vi "ControlsWOOD.vi"() -> ()   [LabVIEW 2016]
uses:
  Typedefs/Sensor Status.ctl
  Modules/Boat/PID Gain.ctl
  Modules/Boat/PID Schedule Entry.ctl
  UI Utilities/ui_states.ctl
  <vilib>/Utility/miscctls.llb/LVPointTypeDef.ctl
  <vilib>/Utility/miscctls.llb/LVPositionTypeDef.ctl
  Messages/autogenerated_vis/receive/mc_receive_state_message.vi
  Minion Core/Minion Core.lvlibp
panel:
  in  "Target":dbl[](array[numeric])
  in  "Main Tabs":T1(tab)
  in  "Navigation Algorithm\nPrimary   -   Fine Manuvering":bool
  out "Back Thrust":dbl(slide) scale=0.0..1.0
  out "?":dbl(slide)
  out "Back Direction":dbl(knob) scale=-1.0..1.0
  out "Front Thrust":dbl(slide) scale=0.0..1.0
  out "?":dbl(slide)
  out "Front Direction":dbl(knob) scale=-1.0..1.0
  in  "Popup Window":bool
  in  "Manage Example":bool
  out "Sensor Status":T2[](array[typedef]) {"Active ID" format="%x"}
  in  "MBED Serial Port":refnum<visa-resource-name>
  out "The String output to mbed":string
  in  "RC(F) Auto(T)":bool
  in  "reinitialize? (F)":bool
  in  "Front Turn Assist Thrust":T3={"Control"={"Mode?"=TRUE, "Active?"=TRUE, "Manual"=0.0}, "PID Schedule"=[], "Input Rate"=0.0, "Output Rate"=0.0, "Filter Input?"=TRUE} {"PID Schedule"."Input Range"."High" format="%.2f"; "PID Schedule"."Input Range"."Low" format="%.2f"; "PID Schedule"."Output Range"."Low" format="%.3f"; "PID Schedule"."Output Range"."High" format="%.3f"; "PID Schedule"."Linearity" format="%#_13g"; "PID Schedule"."PID Gains"."Feedforward"."c" format="%.3f"; "PID Schedule"."PID Gains"."Feedforward"."b" format="%.3f"; "PID Schedule"."PID Gains"."Feedforward"."a" format="%.3f"; "PID Schedule"."PID Gains"."Adv. Gains"."Gamma" format="%.3f"; "PID Schedule"."PID Gains"."Adv. Gains"."Beta" format="%.3f"; "PID Schedule"."PID Gains"."Adv. Gains"."Alpha" format="%.3f"; "PID Schedule"."PID Gains"."Standard Gains"."Kp" format="%.3f"; "PID Schedule"."PID Gains"."Standard Gains"."Ki" format="%.3f"; "PID Schedule"."PID Gains"."Standard Gains"."Kd" format="%.3f"; "Control"."Manual" format="%#_13g"}
  in  "Back Thrust":dbl(slide) scale=0.0..1.0
  in  "Back Steering":T3={"Control"={"Mode?"=TRUE, "Active?"=TRUE, "Manual"=0.0}, "PID Schedule"=[], "Input Rate"=0.0, "Output Rate"=0.0, "Filter Input?"=TRUE} {"PID Schedule"."Input Range"."High" format="%.2f"; "PID Schedule"."Input Range"."Low" format="%.2f"; "PID Schedule"."Output Range"."Low" format="%.3f"; "PID Schedule"."Output Range"."High" format="%.3f"; "PID Schedule"."Linearity" format="%#_13g"; "PID Schedule"."PID Gains"."Feedforward"."c" format="%.3f"; "PID Schedule"."PID Gains"."Feedforward"."b" format="%.3f"; "PID Schedule"."PID Gains"."Feedforward"."a" format="%.3f"; "PID Schedule"."PID Gains"."Adv. Gains"."Gamma" format="%.3f"; "PID Schedule"."PID Gains"."Adv. Gains"."Beta" format="%.3f"; "PID Schedule"."PID Gains"."Adv. Gains"."Alpha" format="%.3f"; "PID Schedule"."PID Gains"."Standard Gains"."Kp" format="%.3f"; "PID Schedule"."PID Gains"."Standard Gains"."Ki" format="%.3f"; "PID Schedule"."PID Gains"."Standard Gains"."Kd" format="%.3f"; "Control"."Manual" format="%#_13g"}
  in  "RC(F) Auto(T)":bool=TRUE
  in  "reinitialize? (F)":bool
  in  "Turbo\nThrust":dbl(slide) scale=0.0..1.0
  in  "Distance\nMinimum for\nTurbo (m)":dbl
  in  "Heading Error\nMaximum for \nTurbo (rad)":dbl
  in  "RC(F) Auto(T)":bool
  in  "reinitialize? (F)":bool
  in  "RC(F) Auto(T)":bool
  in  "reinitialize? (F)":bool
  in  "Desired Boat Orientation":dbl(knob) scale=-180.0..180.0
  in  "Front Thrust":dbl(slide) scale=0.0..1.0
  in  "Back Hold Orientation Thrust":T3={"Control"={"Mode?"=TRUE, "Active?"=TRUE, "Manual"=0.0}, "PID Schedule"=[], "Input Rate"=0.0, "Output Rate"=0.0, "Filter Input?"=TRUE} {"PID Schedule"."Input Range"."High" format="%.2f"; "PID Schedule"."Input Range"."Low" format="%.2f"; "PID Schedule"."Output Range"."Low" format="%.3f"; "PID Schedule"."Output Range"."High" format="%.3f"; "PID Schedule"."Linearity" format="%#_13g"; "PID Schedule"."PID Gains"."Feedforward"."c" format="%.3f"; "PID Schedule"."PID Gains"."Feedforward"."b" format="%.3f"; "PID Schedule"."PID Gains"."Feedforward"."a" format="%.3f"; "PID Schedule"."PID Gains"."Adv. Gains"."Gamma" format="%.3f"; "PID Schedule"."PID Gains"."Adv. Gains"."Beta" format="%.3f"; "PID Schedule"."PID Gains"."Adv. Gains"."Alpha" format="%.3f"; "PID Schedule"."PID Gains"."Standard Gains"."Kp" format="%.3f"; "PID Schedule"."PID Gains"."Standard Gains"."Ki" format="%.3f"; "PID Schedule"."PID Gains"."Standard Gains"."Kd" format="%.3f"; "Control"."Manual" format="%#_13g"}
  in  "Front Eliminate Steering Drift":T3={"Control"={"Mode?"=TRUE, "Active?"=TRUE, "Manual"=0.0}, "PID Schedule"=[], "Input Rate"=0.0, "Output Rate"=0.0, "Filter Input?"=TRUE} {"PID Schedule"."Input Range"."High" format="%.2f"; "PID Schedule"."Input Range"."Low" format="%.2f"; "PID Schedule"."Output Range"."Low" format="%.3f"; "PID Schedule"."Output Range"."High" format="%.3f"; "PID Schedule"."Linearity" format="%#_13g"; "PID Schedule"."PID Gains"."Feedforward"."c" format="%.3f"; "PID Schedule"."PID Gains"."Feedforward"."b" format="%.3f"; "PID Schedule"."PID Gains"."Feedforward"."a" format="%.3f"; "PID Schedule"."PID Gains"."Adv. Gains"."Gamma" format="%.3f"; "PID Schedule"."PID Gains"."Adv. Gains"."Beta" format="%.3f"; "PID Schedule"."PID Gains"."Adv. Gains"."Alpha" format="%.3f"; "PID Schedule"."PID Gains"."Standard Gains"."Kp" format="%.3f"; "PID Schedule"."PID Gains"."Standard Gains"."Ki" format="%.3f"; "PID Schedule"."PID Gains"."Standard Gains"."Kd" format="%.3f"; "Control"."Manual" format="%#_13g"}
  in  "stop":bool
  out "Debug Page":refnum<vi>
  in  "Core Settings":T5={"Communication"={"Interface IP  "="", "Base Port"=50000, "Port Range"=1000}, "Auto Detect "={"Multicast IP"="239.0.0.47", "Multicast Port"=55000, "Heartbeat Timeout (s)"=5.0}, "Logging"={"Max Log Size (MB)"=100, "Log Disk Quota (MB)"=1024, "Minimum Free Space (MB)"=1024, "Log File Directory"=path ""}}
  out "error out":errorcluster
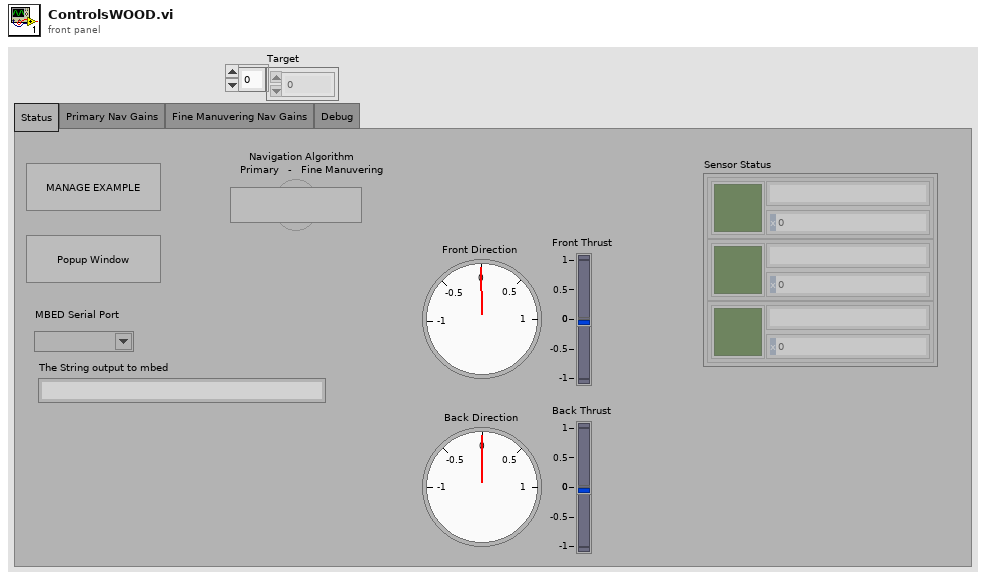
[diagram p1: front panel]
types:
  T1 = enum32{"Status", "Primary Nav Gains", "Fine Manuvering Nav Gains", "Debug"}
  T2 = typedef "Sensor Status.ctl" = cluster{"Status":bool, "Name":string, "Active ID":u8}
  T3 = typedef "PID Gain.ctl" = cluster{"Control":cluster{"Mode?":bool, "Active?":bool, "Manual":dbl}, "PID Schedule":T4[], "Input Rate":dbl, "Output Rate":dbl, "Filter Input?":bool}
  T4 = typedef "PID Schedule Entry.ctl" = cluster{"Schedule Threshold":dbl, "Linearity":dbl, "PID Gains":cluster{"Standard Gains":cluster{"Kp":dbl, "Ki":dbl, "Kd":dbl}, "Adv. Gains":cluster{"Alpha":dbl, "Beta":dbl, "Gamma":dbl}, "Feedforward":cluster{"a":dbl, "b":dbl, "c":dbl}}, "Input Range":cluster{"High":dbl, "Low":dbl}, "Output Range":cluster{"High":dbl, "Low":dbl}}
  T5 = cluster{"Communication":cluster{"Interface IP  ":string, "Base Port":u16, "Port Range":i32}, "Auto Detect ":cluster{"Multicast IP":string, "Multicast Port":u16, "Heartbeat Timeout (s)":dbl}, "Logging":cluster{"Max Log Size (MB)":i64, "Log Disk Quota (MB)":i64, "Minimum Free Space (MB)":i64, "Log File Directory":path}}
  T6 = cluster{"Close Window?":bool, "Example Manager":refnum<vi>, "Popup Example":refnum<vi>}
  T7 = typedef "ui_states.ctl" = enum16{"Setup UI", "Initialize", "Run", "Close"}
  T8 = typedef "state_message.ctl" = cluster{"Global Time Stamp":u64, "NED Time Stamp":u64, "FRD Time Stamp":u64, "Global Position(d)":dbl[], "NED Position (m)":dbl[], "FRD Velocity (m/s)":dbl[], "Rotation Angle (rad)":dbl[], "Angular Rate (rad/s)":dbl[], "NED Error (m)":dbl[], "Velocity Error (m/s)":dbl[], "Angular Error (rad)":dbl[]}
  T9 = typedef "LVPositionTypeDef.ctl" = cluster{"Left":i32, "Top":i32}
  T10 = typedef "LVPointTypeDef.ctl" = cluster{"Horizontal":i16, "Vertical":i16}
  T11 = enum16{"Always On", "Always Off", "Off While Running"}
  T12 = typedef "LVRectTypeDef.ctl" = cluster{"Left":i16, "Top":i16, "Right":i16, "Bottom":i16}
  T13 = typedef "LVBoundsTypeDef.ctl" = cluster{"Width":u32, "Height":u32}
  T14 = cluster{"Shift":bool, "Ctrl":bool, "Alt":bool, "Cmd":bool, "Opt":bool}
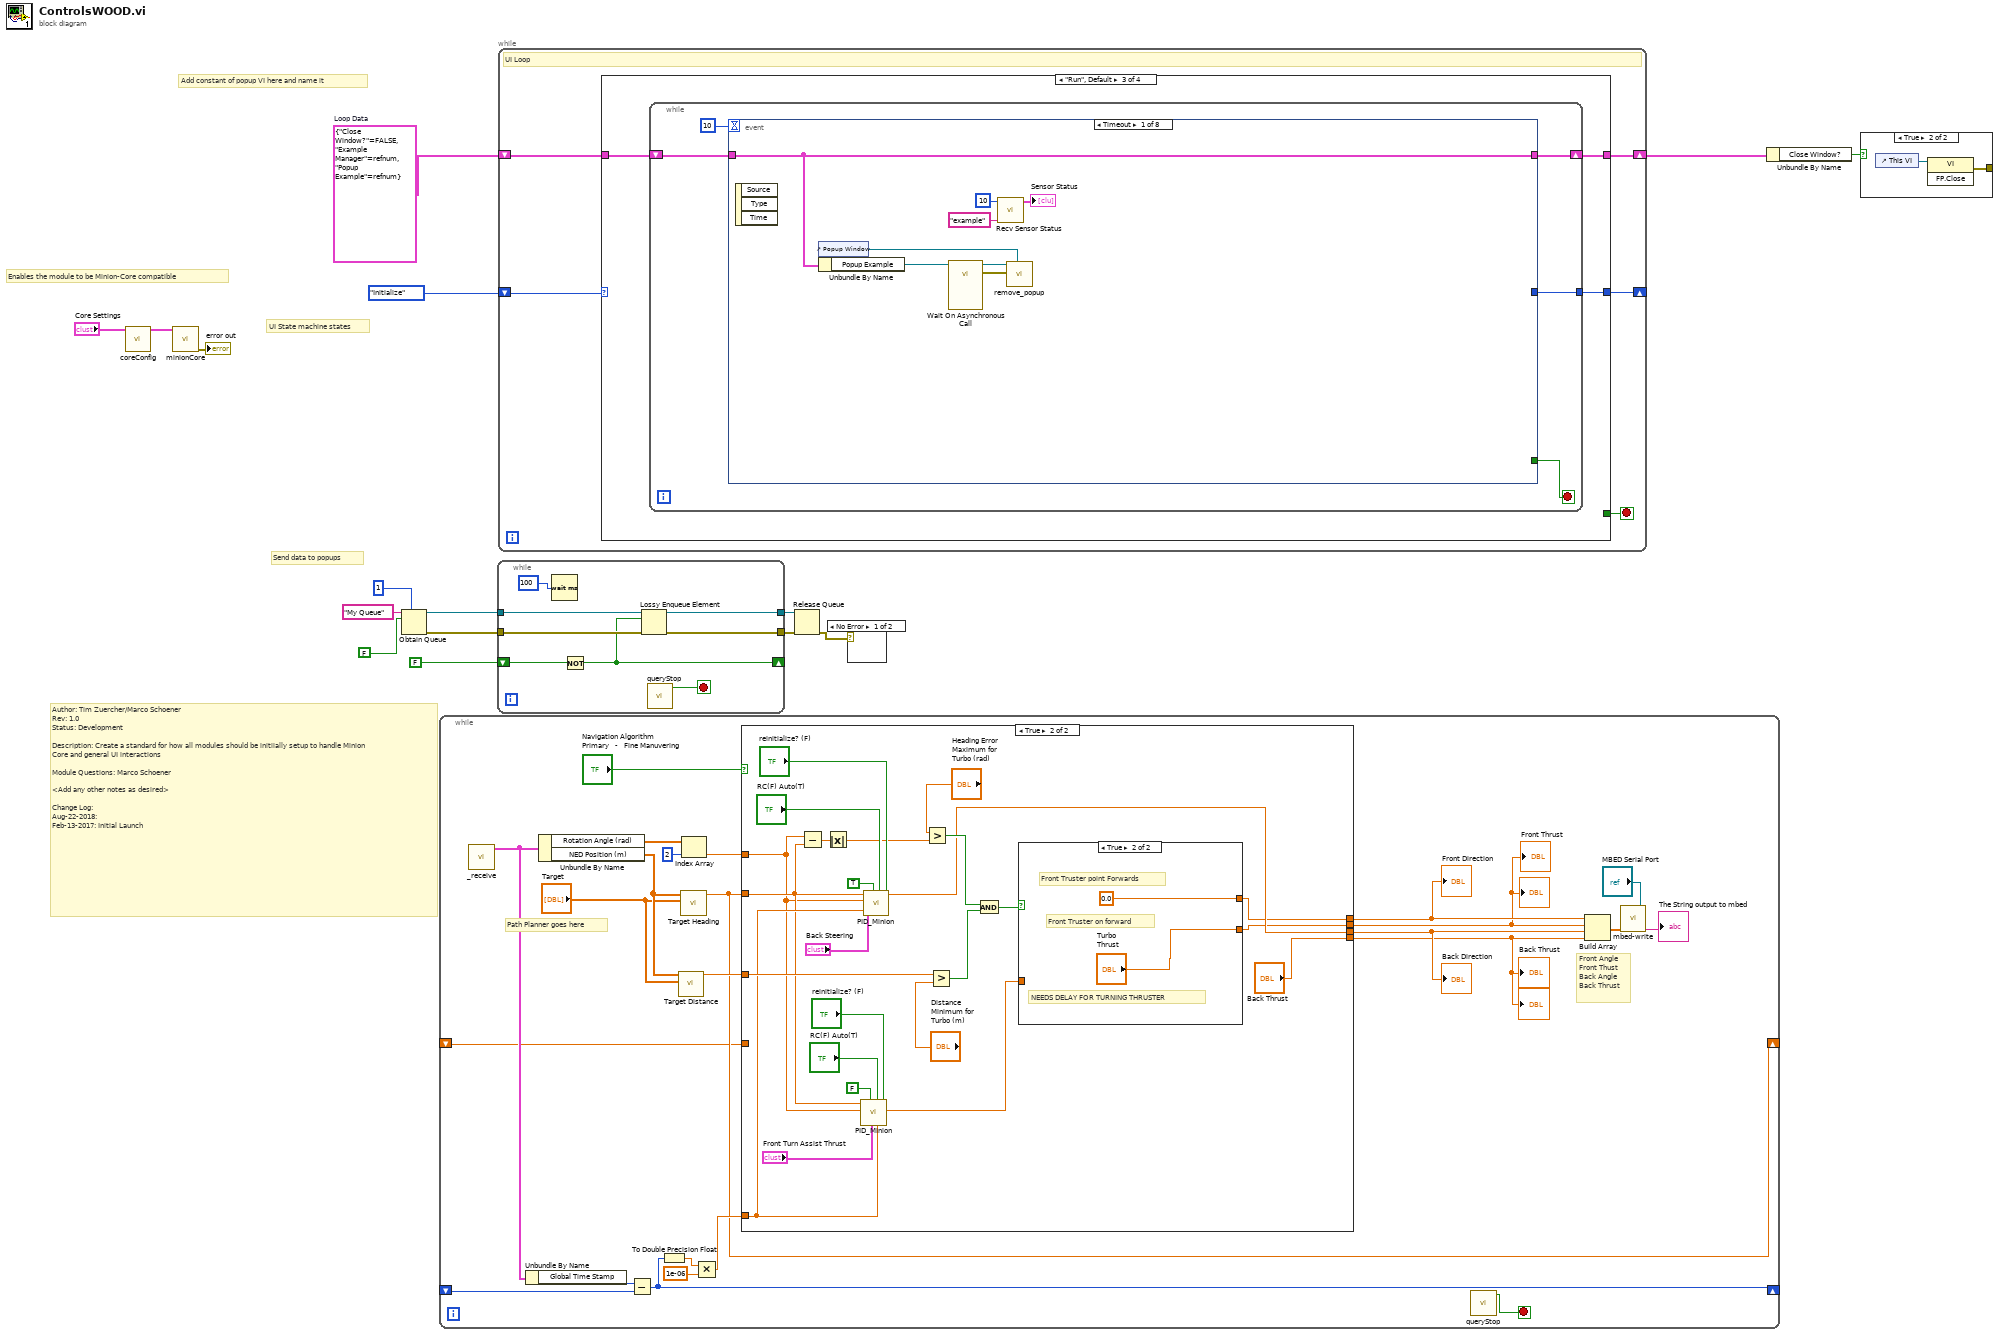
[diagram p0: block diagram]
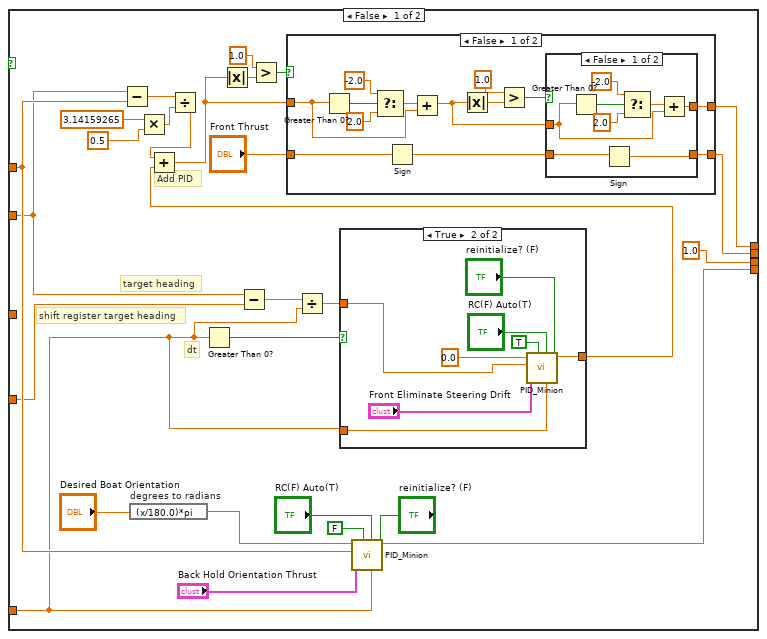
[diagram p2: hidden frame]
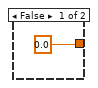
[diagram p3: hidden frame]
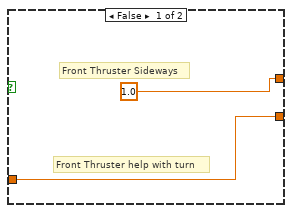
[diagram p6: hidden frame]
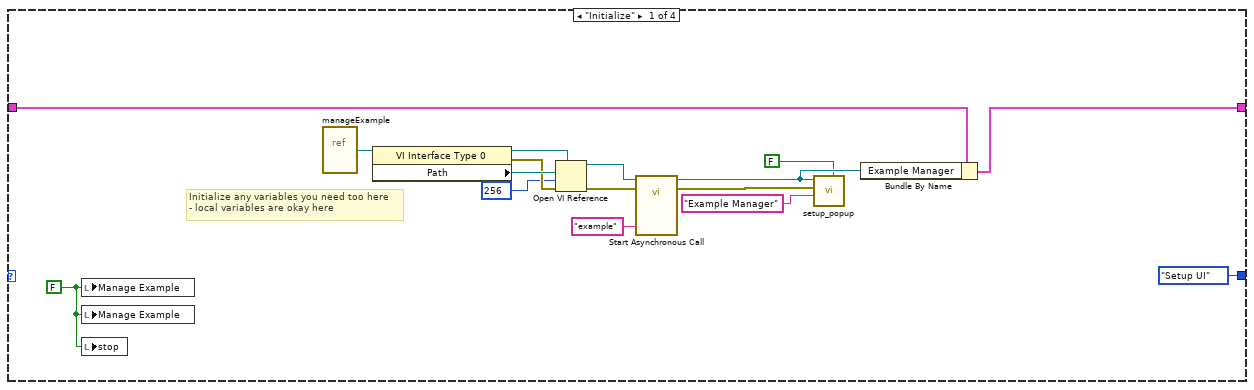
[diagram p9: hidden frame]
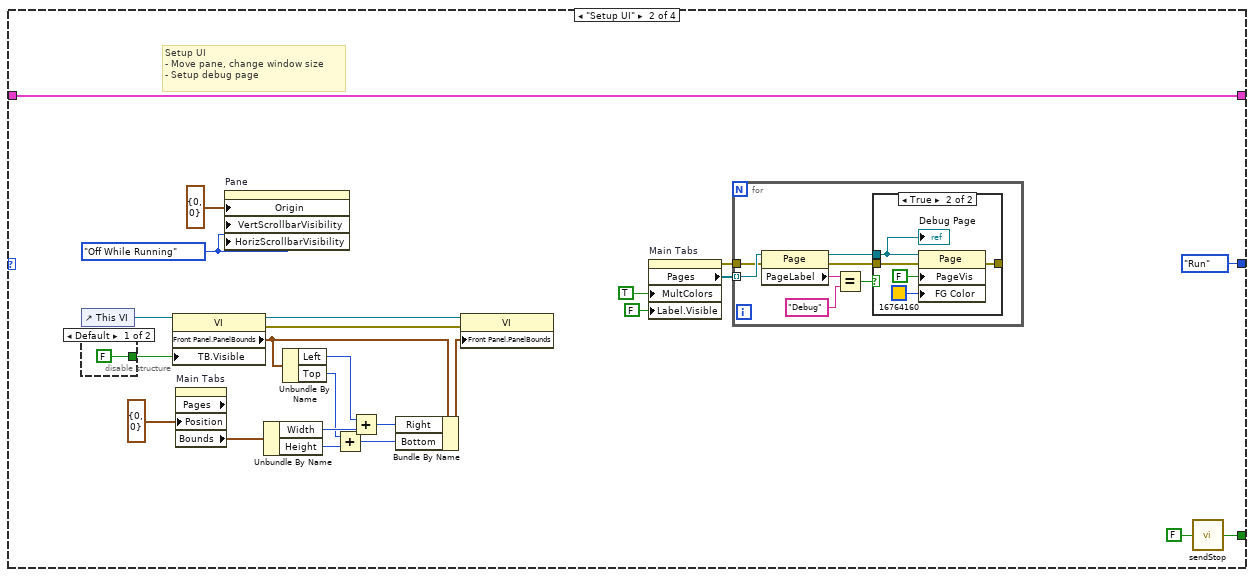
[diagram p10: hidden frame]
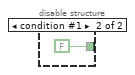
[diagram p11: hidden frame]
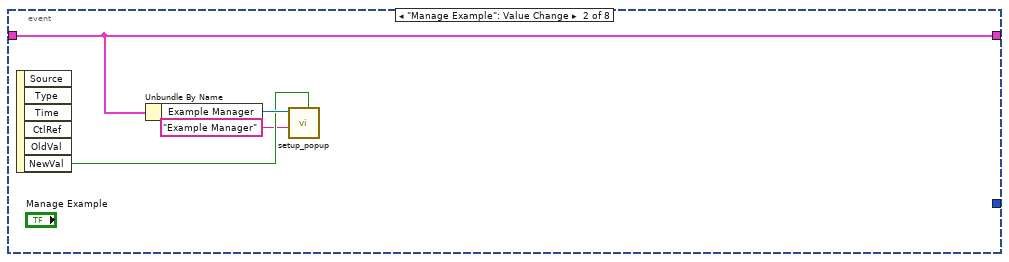
[diagram p13: hidden frame]
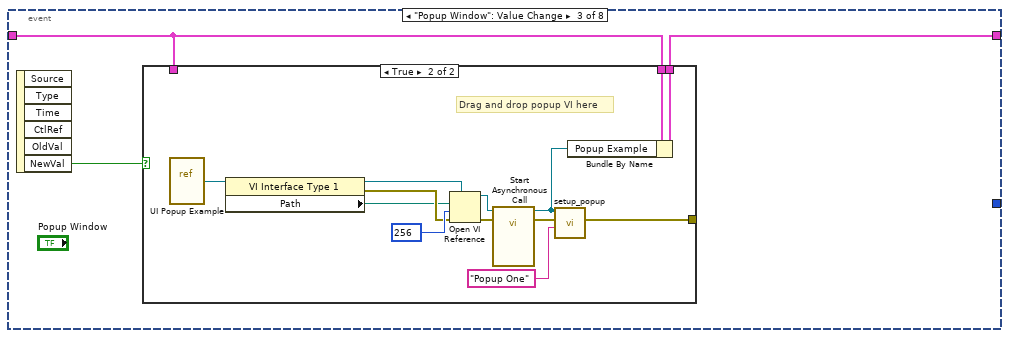
[diagram p14: hidden frame]
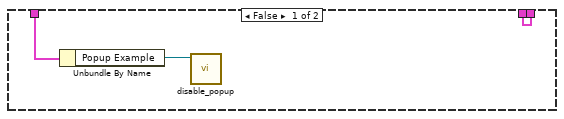
[diagram p15: hidden frame]
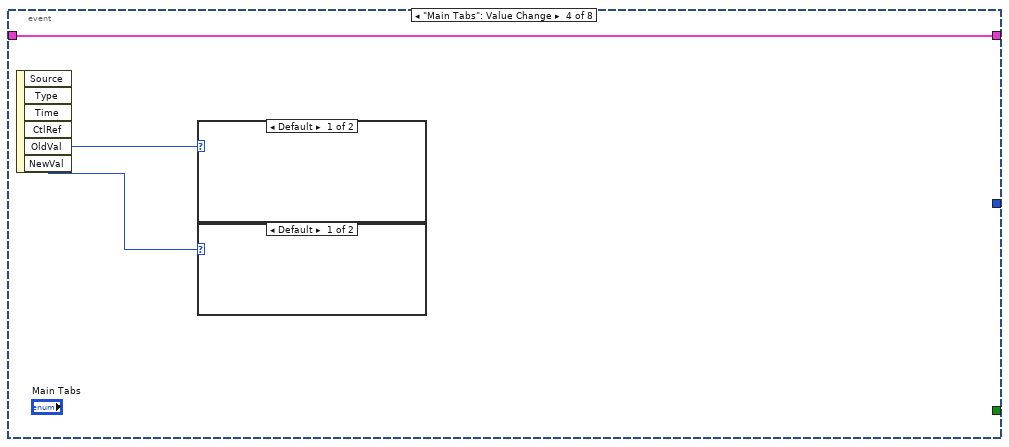
[diagram p16: hidden frame]
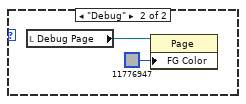
[diagram p17: hidden frame]
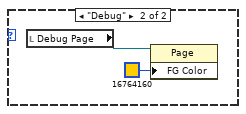
[diagram p18: hidden frame]
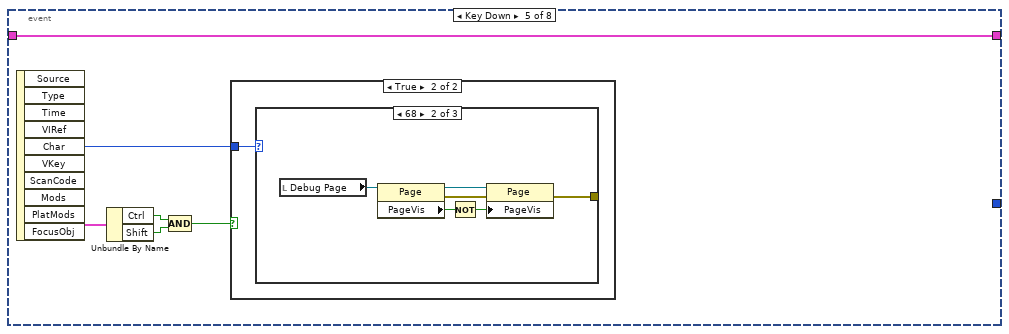
[diagram p19: hidden frame]
diagram:
  w15 = T6 {"Close Window?"=FALSE, "Example Manager"=refnum, "Popup Example"=refnum}  # Loop Data
  # "Author: Tim Zuercher/Marco Schoener\nRev: 1.0\nStatus: Development\n\nDescription: Create a standard for how all modules should be initiially setup to handle Minion Core and general UI interactions\n\nModule Questions: Marco Schoener\n\n<Add any other notes as desired>\n\nChange Log:\nAug-22-2018: \nFeb-13-2017: Initial Launch"
  # "Send data to popups"
  # "Enables the module to be Minion-Core compatible"
  # "UI State machine states"
  # "Add constant of popup VI here and name it"
  n1 = call "coreConfig.vi"("Core Settings"="Core Settings") -> ("Core Settings"=w3:T5)  [unwired: 10 in]
  n2 = call "minionCore.vi"("Core Settings"=w3) -> ("error out"=→"error out":errorcluster)  [unwired: 10 in]
  n3 = Obtain Queue(max queue size (-1, unlimited)=1, name (unnamed)="My Queue", element data type=FALSE) -> (queue out=w13:refnum<queue>, error out=w12:errorcluster)  [unwired: 2 in, 1 out]
  n4 = while {
    shift-right: [w34] -> _
    shift-left: _ -> [w35]
    shift-right: [w18] -> _
    shift-left: _ -> [w17]
    stop <- w40 stop-if-true
    # "Front Angle\nFront Thust\nBack Angle\nBack Thrust"
    # "Path Planner goes here"
    n5 = call-poly "_receive.vi"() -> ("Message"=w37:T8)  [unwired: 7 in, 3 out]
    n6 = Unbundle By Name(w37) -> ("Global Time Stamp"=w36:u64)
    n7 = Unbundle By Name(w37) -> ("Rotation Angle (rad)"=w39:dbl[], "NED Position (m)"=w29:dbl[])
    n8 = Subtract(x=w36, y=w35) -> (x-y=w34:u64)
    n9 = To Double Precision Float(number=w34) -> (double precision float=w33:dbl)
    n10 = call "Target Distance.vi"("Target"="Target", "Position"=w29) -> ("Target Distance"=w27:dbl)  [unwired: 9 in]
    n11 = call "Target Heading.vi"("Target"="Target", "Position"=w29) -> ("Heading (rad)"=w18:dbl)  [unwired: 9 in]
    n12 = Index Array(array=w39, index=2) -> (element=w30:dbl)
    n13 = Multiply(x=w33, y=1e-06) -> (x*y=w31:dbl)
    n14 = case shown="True" "Navigation Algorithm\nPrimary   -   Fine Manuvering" {
      tunnel: w31 -> [w42 w110]
      tunnel: w30 -> [w56 w107]
      tunnel: w18 -> [w48 w108]
      tunnel: w27 -> [_ w120]
      tunnel: [1.0 w114] -> w23
      tunnel: [w45 "Back Thrust"] -> w22
      tunnel: [w60 w112] -> w21
      tunnel: [w59 w111] -> w20
      tunnel: w17 -> [w47 _]
      frame False {
        # "shift register target heading"
        # "target heading"
        # "dt"
        # "Add PID"
        n15 = Subtract(x=w48, y=w56) -> (x-y=w68:dbl)
        n16 = expression code="(x/180.0)*pi" "degrees to radians"("Desired Boat Orientation") -> (w57:dbl)
        n17 = Multiply(x=3.14159265, y=0.5) -> (x*y=w67:dbl)
        n18 = Divide(x=w68, y=w67) -> (x/y=w51:dbl)
        n19 = Greater Than 0?(x=w42) -> (x > 0?=w43:bool)
        n20 = Subtract(x=w48, y=w47) -> (x-y=w46:dbl)
        n21 = Divide(x=w46, y=w42) -> (x/y=w41:dbl)
        n22 = case shown="True" w43 {
          tunnel: [0.0 w72] -> w49
          tunnel: w42 -> [_ w71]
          tunnel: w41 -> [_ w70]
          frame False {
          }
          frame True {
            n23 = call "PID_Minion.vi"("dt (s)"=w71, "RC Auto?"="RC(F) Auto(T)", "reinitialize? (F)"="reinitialize? (F)", "Angle Mode"=TRUE, "PID Gains"="Front Eliminate Steering Drift", "process variable"=w70, "setpoint"=0.0) -> ("output"=w72:dbl)  [unwired: 3 in, 1 out]
          }
        }
        n24 = Add(x=w51, y=w49) -> (x+y=w50:dbl)
        n25 = Absolute Value(x=w50) -> (abs(x)=w62:dbl)
        n26 = Greater?(x=1.0, y=w62) -> (0:w64:bool)
        n27 = case shown="False" w64 {
          tunnel: w50 -> [w86 w102]
          tunnel: [w81 w102] -> w60
          tunnel: [w80 w101] -> w59
          tunnel: "Front Thrust" -> [w79 w101]
          frame False {
            n28 = Greater Than 0?(x=w86) -> (x > 0?=w90:bool)
            n29 = Select(t=-2.0, s=w90, f=2.0) -> (s? t:f=w87:dbl)
            n30 = Sign(1:w79) -> (0:w78:dbl)
            n31 = Add(x=w87, y=w86) -> (x+y=w82:dbl)
            n32 = Absolute Value(x=w82) -> (abs(x)=w84:dbl)
            n33 = Greater?(x=1.0, y=w84) -> (0:w83:bool)
            n34 = case shown="False" w83 {
              tunnel: w82 -> [w95 w100]
              tunnel: [w94 w100] -> w81
              tunnel: w78 -> [w92 w99]
              tunnel: [w91 w99] -> w80
              frame False {
                n35 = Greater Than 0?(x=w95) -> (x > 0?=w98:bool)
                n36 = Sign(1:w92) -> (0:w91:dbl)
                n37 = Select(t=-2.0, s=w98, f=2.0) -> (s? t:f=w96:dbl)
                n38 = Add(x=w96, y=w95) -> (x+y=w94:dbl)
              }
              frame True {
              }
            }
          }
          frame True {
          }
        }
        n39 = call "PID_Minion.vi"("dt (s)"=w42, "RC Auto?"="RC(F) Auto(T)", "reinitialize? (F)"="reinitialize? (F)", "Angle Mode"=FALSE, "PID Gains"="Back Hold Orientation Thrust", "process variable"=w56, "setpoint"=w57) -> ("output"=w45:dbl)  [unwired: 3 in, 1 out]
      }
      frame True {
        n40 = Subtract(x=w107, y=w108) -> (x-y=w115:dbl)
        n41 = Absolute Value(x=w115) -> (abs(x)=w122:dbl)
        n42 = call "PID_Minion.vi"("dt (s)"=w110, "RC Auto?"="RC(F) Auto(T)", "reinitialize? (F)"="reinitialize? (F)", "Angle Mode"=FALSE, "PID Gains"="Front Turn Assist Thrust", "process variable"=w107, "setpoint"=w108) -> ("Setpoint Out"=w103:dbl)  [unwired: 3 in, 1 out]
        n43 = call "PID_Minion.vi"("dt (s)"=w110, "RC Auto?"="RC(F) Auto(T)", "reinitialize? (F)"="reinitialize? (F)", "Angle Mode"=TRUE, "PID Gains"="Back Steering", "process variable"=w107, "setpoint"=w108) -> ("output"=w114:dbl)  [unwired: 3 in, 1 out]
        n44 = Greater?(x="Heading Error\nMaximum for \nTurbo (rad)", y=w122) -> (0:w118:bool)
        n45 = Greater?(x=w120, y="Distance\nMinimum for\nTurbo (m)") -> (0:w117:bool)
        n46 = And(x=w118, y=w117) -> (x .and. y?=w116:bool)
        n47 = case shown="True" w116 {
          tunnel: [1.0 0.0] -> w112
          tunnel: [w127 "Turbo\nThrust"] -> w111
          tunnel: w103 -> [w127 _]
          frame False {
            # "Front Thruster help with turn"
            # "Front Thruster Sideways"
          }
          frame True {
            # "NEEDS DELAY FOR TURNING THRUSTER"
            # "Front Truster on forward"
            # "Front Truster point Forwards"
          }
        }
      }
    }
    "Back Direction" <- w23
    "?" <- w22
    "Back Thrust" <- w22
    "Front Direction" <- w21
    "?" <- w20
    "Front Thrust" <- w20
    n48 = call "queryStop.vi"() -> ("stop?"=w40:bool)  [unwired: 5 in]
    n49 = Build Array(w21, w20, w23, w22) -> (w26:dbl[])
    n50 = call "mbed-write.vi"("Serial Port"="MBED Serial Port", "Array of Numbers"=w26) -> ("Write Output"=→"The String output to mbed":string)  [unwired: 5 in]
  }
  n51 = while {
    tunnel: w13 -> [w137]
    tunnel: w12 -> [w136]
    tunnel: [w135] -> w11
    tunnel: [w134] -> w10
    shift-right: [w131] -> _
    shift-left: FALSE ("element") -> [w132]
    stop <- w138 stop-if-true
    n52 = Wait (ms)(milliseconds to wait=100 ("timeout in ms (-1)")) -> ()  [unwired: 1 out]
    n53 = Not(x=w132) -> (.not. x?=w131:bool)
    n54 = Lossy Enqueue Element(queue=w137, element=w131, error in (no error)=w136) -> (queue out=w134:refnum<queue>, error out=w135:errorcluster)  [unwired: 2 out]
    n55 = call "queryStop.vi"() -> ("stop?"=w138:bool)  [unwired: 5 in]
  }
  n56 = while {
    shift-right: [w142] -> _
    shift-left: ui_states."Initialize" -> [w143]
    shift-right: [w139] -> w1
    shift-left: w15 -> [w140]
    stop <- w141 stop-if-true
    # "UI Loop"
    n57 = case shown="\"Run\", Default" w143 {
      tunnel: [ui_states."Setup UI" ui_states."Run" w200 ui_states."Close"] -> w142
      tunnel: [_ w179 _ w284] -> w141
      tunnel: w140 -> [w146 w160 w199 w271]
      tunnel: [w145 w160 w198 w271] -> w139
      frame "Initialize" {
        w158 = FALSE ("stop")
        # "Initialize any variables you need too here\n- local variables are okay here"
        n58 = local write "Manage Example"(w158) -> ()
        n59 = local write "Manage Example"(w158) -> ()
        n60 = local write "stop"(w158) -> ()
        n61 = vi-ref "manageExample.vi"() -> (w151:refnum<vi>)
        n62 = property class="VI Interface Type 0"(reference=w151) -> (reference out=w155:refnum<vi>, error out=w156:errorcluster, "Path"=w157:path)  [unwired: 1 in]
        n63 = Open VI Reference(type specifier VI Refnum (for type only)=w155, vi path=w157, options=256, error in (no error)=w156) -> (vi reference=w154:refnum<vi>, error out=w153:errorcluster)  [unwired: 2 in]
        n64 = call-by-ref "Start Asynchronous Call"(reference=w154, error in=w153, "Sensor"="example") -> (reference out=w148:refnum<vi>, error out=w149:errorcluster)  [unwired: 11 in]
        n65 = call "setup_popup.vi"("Activate?"=FALSE, "Title"="Example Manager", "error in (no error)"=w149, "reference"=w148) -> ()  [unwired: 7 in, 1 out]
        n66 = Bundle By Name(cluster=w146, "Example Manager"=w148) -> (w145:T6)
      }
      frame "Setup UI" {
        w176 = T11."Off While Running" ("Horizontal Scrollbar Visibility")
        # "Setup UI\n- Move pane, change window size\n- Setup debug page"
        n67 = control-ref of="This VI"() -> (w172:refnum<vi>)
        n68 = disable-structure shown="Default" {
          disable-tunnel: [FALSE ("Label.Visible") FALSE ("Label.Visible")] -> w174
          frame condition #0 (active) {
          }
          frame condition #1 {
          }
        }
        n69 = property class="VI"(reference=w172, "TB.Visible"=w174) -> (reference out=w163:refnum<vi>, error out=w162:errorcluster, "Front Panel.PanelBounds"=w165:T12)  [unwired: 1 in]
        n70 = property on="Main Tabs" class="TabCtl (strict)" props=["Pages", "Position", "Bounds"]("Position"=T9 {"Left"=0, "Top"=0}) -> ("Bounds"=w171:T13)  [unwired: 2 in, 3 out]
        n71 = property on="Pane" class="Pane"("Origin"=T10 {"Horizontal"=0, "Vertical"=0}, "VertScrollbarVisibility"=w176, "HorizScrollbarVisibility"=w176) -> ()  [unwired: 2 in, 2 out]
        n72 = Unbundle By Name(w171) -> ("Width"=w169:u32, "Height"=w167:u32)
        n73 = Unbundle By Name(w165) -> ("Left"=w170:i16, "Top"=w168:i16)
        n74 = Add(x=w168, y=w167) -> (x+y=w161:u32)
        n75 = Add(x=w170, y=w169) -> (x+y=w166:u32)
        n76 = Bundle By Name(cluster=w165, "Right"=w166, "Bottom"=w161) -> (w164:T12)
        n77 = property class="VI"(reference=w163, error in=w162, "Front Panel.PanelBounds"=w164) -> ()  [unwired: 2 out]
        n78 = property on="Main Tabs" class="TabCtl (strict)"("MultColors"=TRUE ("Allow Multiple Colors"), "Label.Visible"=FALSE) -> (error out=w183:errorcluster, "Pages"=w182:refnum<vi>[])  [unwired: 2 in, 1 out]
        n79 = for {
          tunnel: w182 -> [w192] mode=indexing
          tunnel: w183 -> [w186]
          n80 = property class="Page"(reference=w192, error in=w186) -> (reference out=w188:refnum<vi>, error out=w187:errorcluster, "PageLabel"=w191:string)
          n81 = Equal?(x=w191, y="Debug") -> (x = y?=w189:bool)
          n82 = case shown="True" w189 {
            tunnel: w188 -> [_ w196]
            tunnel: w187 -> [_ w195]
            tunnel: [_ w197] -> _
            frame False {
            }
            frame True {
              n83 = property class="Page"(reference=w196, error in=w195, "PageVis"=FALSE ("Page Visible"), "FG Color"=u32 16764160) -> (error out=w197:errorcluster)  [unwired: 1 out]
              "Debug Page" <- w196
            }
          }
        }
        n84 = call "sendStop.vi"("stop"=FALSE) -> ("stop"=w179:bool)  [unwired: 4 in]
      }
      frame "Run", Default {
        n85 = while {
          tunnel: [w204] -> w200
          shift-right: [w201] -> w198
          shift-left: w199 -> [w202]
          stop <- w205 stop-if-true
          n86 = event shown="[0] Timeout" {
            selector: _ -> [_ _ _ _ _ _ _ _]
            dyn-events: _ -> [_ _ _ _ _ _ _ _]
            timeout: 10 -> [_ _ _ _ _ _ _ _]
            tunnel: [_ _ _ _ _ _ _ w267] -> w205
            tunnel: [_ _ _ _ _ ui_states."Close" ui_states."Close" w268] -> w204
            tunnel: w202 -> [w209 w216 w218 w237 w244 w260 w263 w266]
            tunnel: [w209 w216 w219 w237 w244 w259 w263 w266] -> w201
            event Timeout {
              n87 = event-data() -> ()  [unwired: 1 in, 3 out]
              n88 = control-ref of="Popup Window"() -> (w206:refnum<vi>)
              n89 = Unbundle By Name(w209) -> ("Popup Example"=w208:refnum<vi>)
              n90 = call-by-ref "Wait On Asynchronous Call"(reference=w208) -> (reference out=w207:refnum<vi>, error out=w210:errorcluster)  [unwired: 13 in]
              n91 = call "Recv Sensor Status.vi"("Sensor Name"="example", "Timeout"=10) -> ("Sensor Status"=→"Sensor Status":T2[])  [unwired: 8 in, 1 out]
              n92 = call "remove_popup.vi"("Button Reference"=w206, "error in (no error)"=w210, "VI Reference"=w207) -> ()  [unwired: 9 in]
            }
            event "Manage Example": Value Change {
              n93 = event-data() -> ("NewVal"=w215:bool)  [unwired: 1 in, 5 out]
              n94 = Unbundle By Name(w216) -> ("Example Manager"=w217:refnum<vi>)
              n95 = call "setup_popup.vi"("Activate?"=w215, "Title"="Example Manager", "reference"=w217) -> ()  [unwired: 8 in, 1 out]
            }
            event "Popup Window": Value Change {
              n96 = event-data() -> ("NewVal"=w220:bool)  [unwired: 1 in, 5 out]
              n97 = case shown="True" w220 {
                tunnel: w218 -> [w221 w234]
                tunnel: [w221 w233] -> w219
                tunnel: [_ w230] -> _
                tunnel: w218 -> [w223 _]
                frame False {
                  n98 = Unbundle By Name(w223) -> ("Popup Example"=w222:refnum<vi>)
                  n99 = call "disable_popup.vi"("reference"=w222) -> ()  [unwired: 10 in]
                }
                frame True {
                  # "Drag and drop popup VI here"
                  n100 = vi-ref "UI Popup Example.vi"() -> (w227:refnum<vi>)
                  n101 = property class="VI Interface Type 1"(reference=w227) -> (reference out=w226:refnum<vi>, error out=w225:errorcluster, "Path"=w224:path)  [unwired: 1 in]
                  n102 = Open VI Reference(type specifier VI Refnum (for type only)=w226, vi path=w224, options=256, error in (no error)=w225) -> (vi reference=w232:refnum<vi>, error out=w236:errorcluster)  [unwired: 2 in]
                  n103 = call-by-ref "Start Asynchronous Call"(reference=w232, error in=w236) -> (reference out=w229:refnum<vi>, error out=w231:errorcluster)  [unwired: 12 in]
                  n104 = call "setup_popup.vi"("Title"="Popup One", "error in (no error)"=w231, "reference"=w229) -> ("error out"=w230:errorcluster)  [unwired: 8 in]
                  n105 = Bundle By Name(cluster=w234, "Popup Example"=w229) -> (w233:T6)
                }
              }
            }
            event "Main Tabs": Value Change {
              n106 = event-data() -> ("OldVal"=w239:T1, "NewVal"=w238:T1)  [unwired: 1 in, 4 out]
              n107 = case shown="Default" w239 {
                frame Default {
                }
                frame "Debug" {
                  n108 = local read "Debug Page"() -> (w242:refnum<vi>)
                  n109 = property class="Page"(reference=w242, "FG Color"=u32 16764160) -> ()  [unwired: 1 in, 2 out]
                }
              }
              n110 = case shown="Default" w238 {
                frame Default {
                }
                frame "Debug" {
                  n111 = local read "Debug Page"() -> (w240:refnum<vi>)
                  n112 = property class="Page"(reference=w240, "FG Color"=u32 11776947) -> ()  [unwired: 1 in, 2 out]
                }
              }
            }
            event Key Down {
              n113 = event-data() -> ("Char"=w246:i16, "PlatMods"=w249:T14)  [unwired: 1 in, 8 out]
              n114 = Unbundle By Name(w249) -> ("Ctrl"=w248:bool, "Shift"=w247:bool)
              n115 = Compound Arithmetic op=AND(w248, w247) -> (w245:bool)
              n116 = case shown="True" w245 {
                tunnel: w246 -> [_ w250]
                frame False {
                }
                frame True {
                  n117 = case shown="68" w250 {
                    tunnel: [_ w252 _] -> _
                    frame Default {
                    }
                    frame 68 {
                      n118 = local read "Debug Page"() -> (w251:refnum<vi>)
                      n119 = property class="Page"(reference=w251) -> (reference out=w255:refnum<vi>, error out=w256:errorcluster, "PageVis"=w254:bool)  [unwired: 1 in]
                      n120 = Not(x=w254) -> (.not. x?=w253:bool)
                      n121 = property class="Page"(reference=w255, error in=w256, "PageVis"=w253) -> (error out=w252:errorcluster)  [unwired: 1 out]
                    }
                    frame 81 {
                      n122 = property on="stop" class="Bool (strict)"("Val(Sgnl)"=TRUE ("Value (Signaling)")) -> ()  [unwired: 2 in, 2 out]
                    }
                  }
                }
              }
            }
            event Panel Close? {
              w258 = TRUE ("Close Window?")
              n123 = event-data() -> ()  [unwired: 1 in, 4 out]
              n124 = property on="stop" class="Bool (strict)"("Val(Sgnl)"=TRUE ("Value (Signaling)")) -> ()  [unwired: 2 in, 2 out]
              n125 = Bundle By Name(cluster=w260, "Close Window?"=w258) -> (w259:T6)
              n126 = event-data("Discard?"=w258) -> ()  [unwired: 1 in, 1 out]
            }
            event Application Instance Close {
              n127 = event-data() -> ()  [unwired: 1 in, 4 out]
              n128 = property on="stop" class="Bool (strict)"("Val(Sgnl)"=TRUE ("Value (Signaling)")) -> ()  [unwired: 2 in, 2 out]
            }
            event "stop": Value Change {
              n129 = event-data() -> ("NewVal"=w267:bool)  [unwired: 1 in, 5 out]
              n130 = case shown="True" w267 {
                tunnel: [ui_states."Run" ui_states."Close"] -> w268
                frame False {
                }
                frame True {
                }
              }
            }
          }
        }
      }
      frame "Close" {
        # "Give popups time to close normally beofre forcing them closed"
        # "Call minion core stop"
        # "Destroy anything you need to here\n- Close popups\n- Close files/logs"
        n131 = control-ref of="Manage Example"() -> (w282:refnum<vi>)
        n132 = Unbundle By Name(w271) -> ("Example Manager"=w283:refnum<vi>)
        n133 = control-ref of="Popup Window"() -> (w273:refnum<vi>)
        n134 = Unbundle By Name(w271) -> ("Popup Example"=w272:refnum<vi>)
        n135 = flat-sequence {
          tunnel: w283 -> [w293]
          tunnel: w282 -> [w294]
          tunnel: [w293] -> w280
          tunnel: [w294] -> w279
          tunnel: [w296] -> w281
          tunnel: w280 -> [w296]
          tunnel: w279 -> [w295]
          tunnel: [w295] -> w278
          tunnel: w281 -> [w299]
          tunnel: w278 -> [w298]
          frame #0 {
            n136 = call "disable_popup.vi"("reference"=w293) -> ()  [unwired: 10 in]
          }
          frame #1 {
            n137 = Wait (ms)(milliseconds to wait=u32 1000) -> ()  [unwired: 1 out]
          }
          frame #2 {
            n138 = call "remove_popup.vi"("Button Reference"=w298, "VI Reference"=w299) -> ()  [unwired: 10 in]
          }
        }
        n139 = flat-sequence {
          tunnel: w272 -> [w286]
          tunnel: w273 -> [w287]
          tunnel: [w286] -> w277
          tunnel: [w287] -> w276
          tunnel: [w289] -> w275
          tunnel: w277 -> [w289]
          tunnel: w276 -> [w288]
          tunnel: [w288] -> w274
          tunnel: w275 -> [w292]
          tunnel: w274 -> [w291]
          frame #0 {
            n140 = call "disable_popup.vi"("reference"=w286) -> ()  [unwired: 10 in]
          }
          frame #1 {
            n141 = Wait (ms)(milliseconds to wait=u32 100) -> ()  [unwired: 1 out]
          }
          frame #2 {
            n142 = call "remove_popup.vi"("Button Reference"=w291, "VI Reference"=w292) -> ()  [unwired: 10 in]
          }
        }
        n143 = while {
          tunnel: [w300] -> w284
          stop <- w300 stop-if-true
          n144 = call "sendStop.vi"("stop"=TRUE) -> ("stop"=w300:bool)  [unwired: 4 in]
        }
      }
    }
  }
  n145 = Release Queue(queue=w10, error in (no error)=w11) -> (error out=w9:errorcluster)  [unwired: 1 in, 2 out]
  n146 = case shown="No Error" w9 {
    frame No Error {
    }
    frame Error {
    }
  }
  n147 = Unbundle By Name(w1) -> ("Close Window?"=w2:bool)
  n148 = case shown="True" w2 {
    tunnel: [_ w302] -> _
    frame False {
    }
    frame True {
      n149 = control-ref of="This VI"() -> (w303:refnum<vi>)
      n150 = invoke class="VI" method="FP.Close"(reference=w303) -> (error out=w302:errorcluster)  [unwired: 2 in, 2 out]
    }
  }
